vi "VersionStrings.Get.vi"(8 "error in (no error)":errorcluster, 11 "Version Build Information":T1={"VeriStand Version"="2013 SP1", "TestStand Version"="2013", "New VS Assembly Version"="2013.0.0.0", "New TS Assembly Version"="5.1.0.226", "VeriStand Steps Version String"="14.0.5.0", "Project Paths"={"MiscHelperVIs Project Path"="", "RTSequenceVIs Project Path"="", "Set Channels Project Path"="", "TS VS Logger Project Path"="", "VeriStand.exe Install Path"="", "NI_VeristandTypes.ini File Path"="", "Workspace Path"="", "VeristandSteps.csproj File Path"="", "Silent Veristand Project Path"=""}, "New TS Interop Assembly Version"="1.2.3.4", "New TS Utility Assembly Version"="5.6.7.8", "New VS Assembly Version (GAC)"="4.0.2016.0.9.9", "dotNET .config File Paths"={"MiscHelperVIs Project .config File Path"=path "C:/Users/Public/Documents/Git-Source/VeriStand-Custom-Steps-For-TestStand/Source/LabVIEW Code/Misc/MiscHelperVIs.lvproj.config", "RT Sequence VIs Project .config File Path"=path "C:/Users/Public/Documents/Git-Source/VeriStand-Custom-Steps-For-TestStand/Source/LabVIEW Code/RT Sequence/RTSequenceVIs.lvproj.config", "Set Channels Project .config File Path"=path "C:/Users/Public/Documents/Git-Source/VeriStand-Custom-Steps-For-TestStand/Source/LabVIEW Code/Set Channels/Set Channels.lvproj.config", "TS VS Logger Project .config File Path"=path "C:/Users/Public/Documents/Git-Source/VeriStand-Custom-Steps-For-TestStand/Source/LabVIEW Code/TS VS Logger/TS VS Logger.lvproj.config", "Silent Veristand Project .config File Path"=path "C:/Users/Public/Documents/Git-Source/VeriStand-Custom-Steps-For-TestStand/Source/LabVIEW Code/VeriStand Silent Start/SilentVS.lvproj.config"}}) -> (0 "error out":errorcluster, 3 "Version Build Information out":T1={"VeriStand Version"="2013 SP1", "TestStand Version"="2013", "New VS Assembly Version"="2013.0.0.0", "New TS Assembly Version"="5.1.0.226", "VeriStand Steps Version String"="14.0.5.0", "Project Paths"={"MiscHelperVIs Project Path"="", "RTSequenceVIs Project Path"="", "Set Channels Project Path"="", "TS VS Logger Project Path"="", "VeriStand.exe Install Path"="", "NI_VeristandTypes.ini File Path"="", "Workspace Path"="", "VeristandSteps.csproj File Path"="", "Silent Veristand Project Path"=""}, "New TS Interop Assembly Version"="1.2.3.4", "New TS Utility Assembly Version"="5.6.7.8", "New VS Assembly Version (GAC)"="4.0.2016.0.9.9", "dotNET .config File Paths"={"MiscHelperVIs Project .config File Path"=path "C:/Users/Public/Documents/Git-Source/VeriStand-Custom-Steps-For-TestStand/Source/LabVIEW Code/Misc/MiscHelperVIs.lvproj.config", "RT Sequence VIs Project .config File Path"=path "C:/Users/Public/Documents/Git-Source/VeriStand-Custom-Steps-For-TestStand/Source/LabVIEW Code/RT Sequence/RTSequenceVIs.lvproj.config", "Set Channels Project .config File Path"=path "C:/Users/Public/Documents/Git-Source/VeriStand-Custom-Steps-For-TestStand/Source/LabVIEW Code/Set Channels/Set Channels.lvproj.config", "TS VS Logger Project .config File Path"=path "C:/Users/Public/Documents/Git-Source/VeriStand-Custom-Steps-For-TestStand/Source/LabVIEW Code/TS VS Logger/TS VS Logger.lvproj.config", "Silent Veristand Project .config File Path"=path "C:/Users/Public/Documents/Git-Source/VeriStand-Custom-Steps-For-TestStand/Source/LabVIEW Code/VeriStand Silent Start/SilentVS.lvproj.config"}})   [LabVIEW 2014, in "VeriStand Steps Version Mutation.lvlib"]
uses:
  VeriStand Steps Version Mutation.lvlib
  Types/Version Build Information.ctl
  Types/Project Paths Cluster.ctl
  Types/dotNET Config File Paths Cluster.ctl
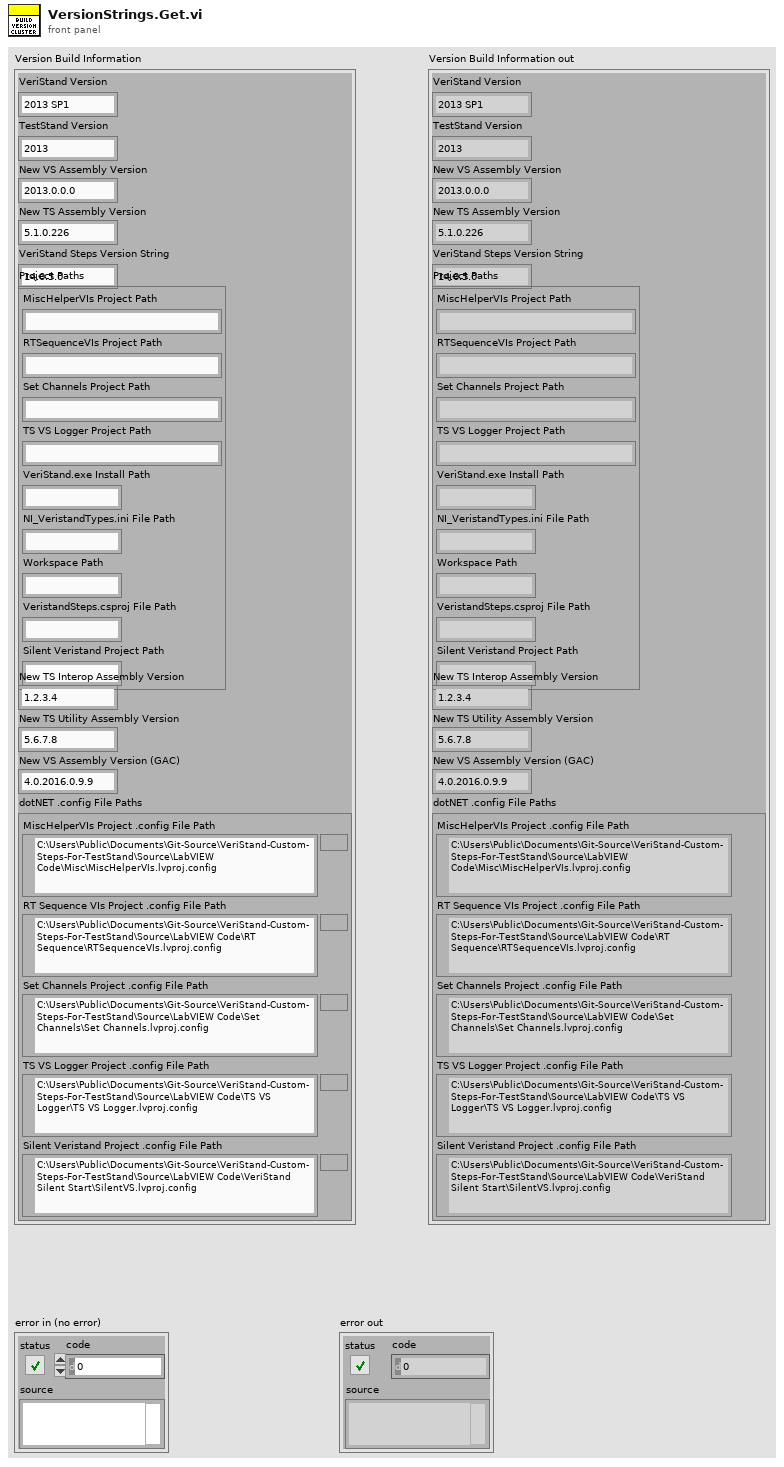
[diagram p1: front panel]
types:
  T1 = typedef "VeriStand Steps Version Mutation.lvlib/Version Build Information.ctl" = cluster{"VeriStand Version":string, "TestStand Version":string, "New VS Assembly Version":string, "New TS Assembly Version":string, "VeriStand Steps Version String":string, "Project Paths":T2, "New TS Interop Assembly Version":string, "New TS Utility Assembly Version":string, "New VS Assembly Version (GAC)":string, "dotNET .config File Paths":T3}
  T2 = typedef "VeriStand Steps Version Mutation.lvlib/Project Paths Cluster.ctl" = cluster{"MiscHelperVIs Project Path":string, "RTSequenceVIs Project Path":string, "Set Channels Project Path":string, "TS VS Logger Project Path":string, "VeriStand.exe Install Path":string, "NI_VeristandTypes.ini File Path":string, "Workspace Path":string, "VeristandSteps.csproj File Path":string, "Silent Veristand Project Path":string}
  T3 = typedef "VeriStand Steps Version Mutation.lvlib/dotNET Config File Paths Cluster.ctl" = cluster{"MiscHelperVIs Project .config File Path":path, "RT Sequence VIs Project .config File Path":path, "Set Channels Project .config File Path":path, "TS VS Logger Project .config File Path":path, "Silent Veristand Project .config File Path":path}
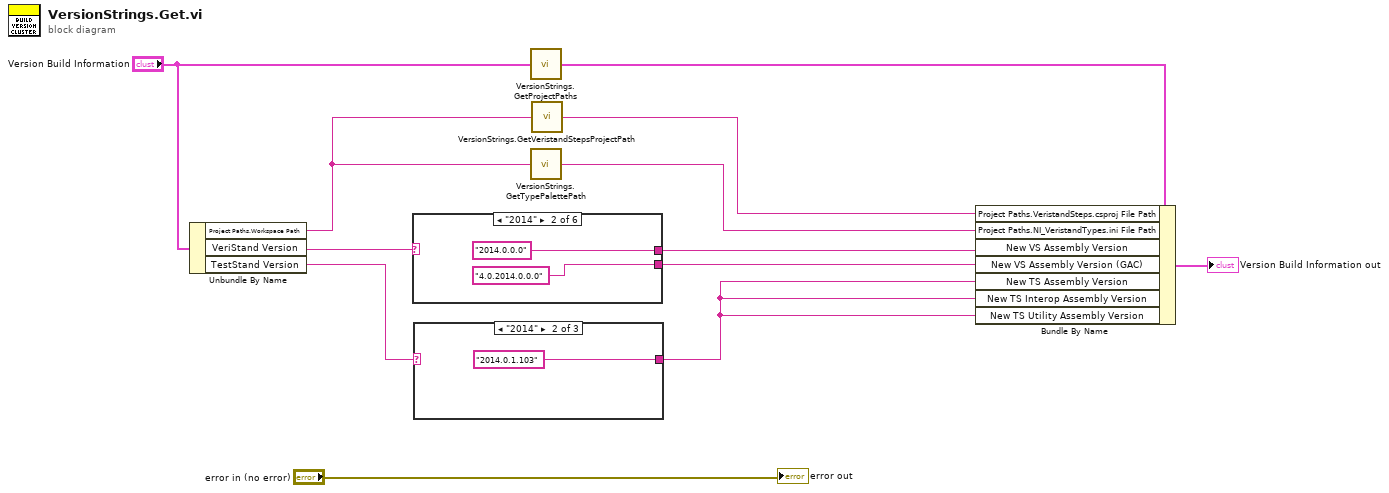
[diagram p0: block diagram]
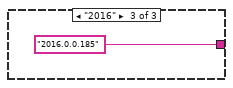
[diagram p3: hidden frame]
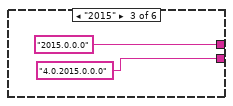
[diagram p5: hidden frame]
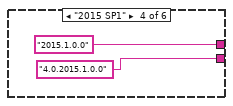
[diagram p6: hidden frame]
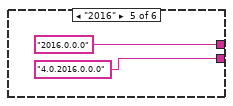
[diagram p7: hidden frame]
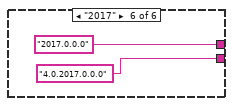
[diagram p8: hidden frame]
diagram:
  n1 = Unbundle By Name("Version Build Information") -> ("Project Paths.Workspace Path"=w5:string, "VeriStand Version"=w11:string, "TestStand Version"=w10:string)
  n2 = case shown="\"2014\"" w11 {
    tunnel: [_ "2014.0.0.0" "2015.0.0.0" "2015.1.0.0" "2016.0.0.0" "2017.0.0.0"] -> w9
    tunnel: [_ "4.0.2014.0.0.0" "4.0.2015.0.0.0" "4.0.2015.1.0.0" "4.0.2016.0.0.0" "4.0.2017.0.0.0"] -> w8
    frame "False", Default {
    }
    frame "2014" {
    }
    frame "2015" {
    }
    frame "2015 SP1" {
    }
    frame "2016" {
    }
    frame "2017" {
    }
  }
  n3 = case shown="\"2014\"" w10 {
    tunnel: [_ "2014.0.1.103" "2016.0.0.185"] -> w7
    frame "False", Default {
    }
    frame "2014" {
    }
    frame "2016" {
    }
  }
  n4 = call "VersionStrings.GetProjectPaths.vi"("Version Build Info"="Version Build Information") -> ("Version Build Info out"=w2:T1)
  n5 = call "VersionStrings.GetTypePalettePath.vi"("Workspace Path"=w5) -> ("NI_VeristandTypes.ini File Path"=w6:string)
  n6 = call "VersionStrings.GetVeristandStepsProjectPath.vi"("Workspace Path"=w5) -> ("VeristandSteps.csproj File Path"=w4:string)
  n7 = Bundle By Name(cluster=w2, "Project Paths.VeristandSteps.csproj File Path"=w4, "Project Paths.NI_VeristandTypes.ini File Path"=w6, "New VS Assembly Version"=w9, "New VS Assembly Version (GAC)"=w8, "New TS Assembly Version"=w7, "New TS Interop Assembly Version"=w7, "New TS Utility Assembly Version"=w7) -> (→"Version Build Information out":T1)
  "error out" <- "error in (no error)"
